vi "CreateRampTask.vi"(8 "error in":errorcluster, 9 "sample mode":i32(ring)=10123 items=["Finite Samples"=10178, "Continuous Samples"=10123, "Hardware Timed Single Point"=12522], 10 "Sample Rate":dbl=1000.0 format="%0.2f", 11 "Number of Samples":i32=1) -> (0 "error out":errorcluster, 3 "task out":refnum<k21>)   [LabVIEW 2015]
uses:
  <vilib>/DAQmx/configure/timing.llb/DAQmx Timing (Sample Clock).vi
  <vilib>/DAQmx/create/channels.llb/DAQmx Create Channel (AO-Voltage-Basic).vi
  <resource>/objmgr/daqmx.rc
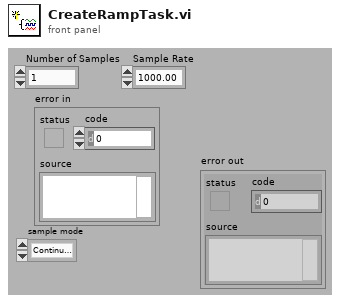
[diagram p1: front panel]
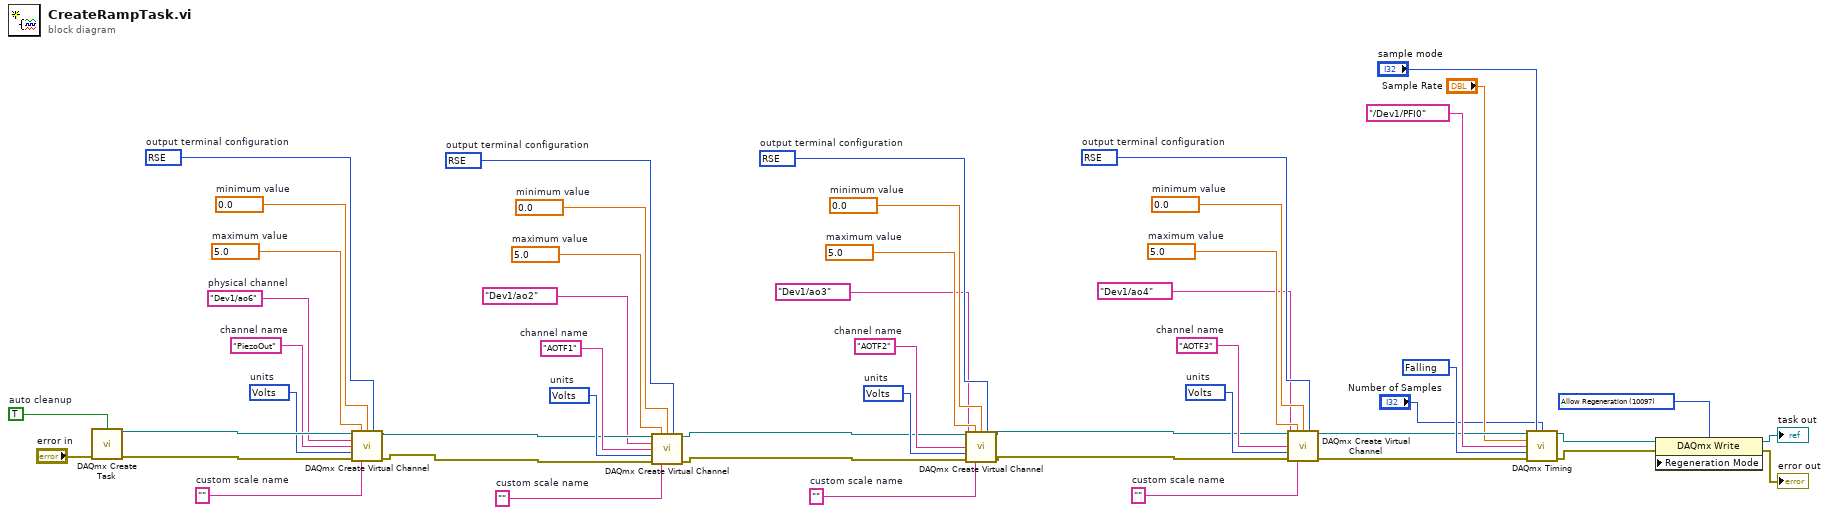
[diagram p0: block diagram]
diagram:
  w5 = 10097 items=["Allow Regeneration"=10097, "Do Not Allow Regeneration"=10158] ("RegenMode")
  w14 = 10083 items=["Default"=-1, "RSE"=10083, "Differential"=10106, "Pseudodifferential"=12529]  # output terminal configuration
  w15 = 10348 items=["Volts"=10348, "From Custom Scale"=10065]  # units
  w16 = "AOTF3"  # channel name
  w17 = ""  # custom scale name
  w18 = 0.0  # minimum value
  w19 = 5.0  # maximum value
  w23 = 10083 items=["Default"=-1, "RSE"=10083, "Differential"=10106, "Pseudodifferential"=12529]  # output terminal configuration
  w24 = 10348 items=["Volts"=10348, "From Custom Scale"=10065]  # units
  w25 = "AOTF2"  # channel name
  w26 = ""  # custom scale name
  w27 = 0.0  # minimum value
  w28 = 5.0  # maximum value
  w31 = 10083 items=["Default"=-1, "RSE"=10083, "Differential"=10106, "Pseudodifferential"=12529]  # output terminal configuration
  w32 = 10348 items=["Volts"=10348, "From Custom Scale"=10065]  # units
  w33 = "AOTF1"  # channel name
  w34 = ""  # custom scale name
  w35 = 0.0  # minimum value
  w36 = 5.0  # maximum value
  w38 = 10171 items=["Rising"=10280, "Falling"=10171] ("active edge")
  w40 = 10083 items=["Default"=-1, "RSE"=10083, "Differential"=10106, "Pseudodifferential"=12529]  # output terminal configuration
  w41 = 10348 items=["Volts"=10348, "From Custom Scale"=10065]  # units
  w42 = "PiezoOut"  # channel name
  w43 = ""  # custom scale name
  w44 = 0.0  # minimum value
  w45 = 5.0  # maximum value
  w46 = "Dev1/ao6"  # physical channel
  w48 = TRUE  # auto cleanup
  n1 = call <vilib>:"DAQmx Create Task.vi"("auto cleanup"=w48, "error in"="error in") -> ("task out"=w47:refnum<k21>, "error out"=w49:errorcluster)  [unwired: 12 in]
  n2 = call-poly <vilib>:"DAQmx Create Virtual Channel.vi"("task in"=w47, "maximum value"=w45, "minimum value"=w44, "output terminal configuration"=w40, "physical channels"=w46, "name to assign"=w42, "units"=w41, "error in"=w49, "custom scale name"=w43) -> ("task out"=w30:refnum<k21>, "error out"=w29:errorcluster)  [unwired: 5 in]
  n3 = call-poly <vilib>:"DAQmx Create Virtual Channel.vi"("task in"=w30, "maximum value"=w36, "minimum value"=w35, "output terminal configuration"=w31, "physical channels"=tag "Dev1/ao2", "name to assign"=w33, "units"=w32, "error in"=w29, "custom scale name"=w34) -> ("task out"=w22:refnum<k21>, "error out"=w21:errorcluster)  [unwired: 5 in]
  n4 = call-poly <vilib>:"DAQmx Create Virtual Channel.vi"("task in"=w22, "maximum value"=w28, "minimum value"=w27, "output terminal configuration"=w23, "physical channels"=tag "Dev1/ao3", "name to assign"=w25, "units"=w24, "error in"=w21, "custom scale name"=w26) -> ("task out"=w12:refnum<k21>, "error out"=w11:errorcluster)  [unwired: 5 in]
  n5 = call-poly <vilib>:"DAQmx Create Virtual Channel.vi"("task in"=w12, "maximum value"=w19, "minimum value"=w18, "output terminal configuration"=w14, "physical channels"=tag "Dev1/ao4", "name to assign"=w16, "units"=w15, "error in"=w11, "custom scale name"=w17) -> ("task out"=w10:refnum<k21>, "error out"=w9:errorcluster)  [unwired: 5 in]
  n6 = call-poly <vilib>:"DAQmx Timing.vi"("task/channels in"=w10, "sample mode"="sample mode", "samples per channel"="Number of Samples", "rate"="Sample Rate", "source"=tag "/Dev1/PFI0", "active edge"=w38, "error in"=w9) -> ("task out"=w7:refnum<k21>, "error out"=w6:errorcluster)  [unwired: 7 in]
  n7 = property class="DAQmx Write"(reference=w7, error in=w6, "Regeneration Mode"=w5) -> (reference out=→"task out":refnum<k21>, error out=→"error out":errorcluster)
